vi "Morphological Segmentation.vi"() -> ()   [LabVIEW 2014]
doc: "This example demonstrates a watershed transform as part of a morphological segmentation process. First, a sample image is thesholded, and a distance transform is applied to the sample image. Next, a watershed transform is applied to the image. A threshold of the watershed image is then used to separate the particles."
uses:
  <vilib>/vision/NI_Vision_Development_Module.lvlib
panel:
  in  "Images":T1(tab)=enum."Result Image"
  out "Source Image":T2(plugin-control)
  out "Threshold Image":T2(plugin-control)
  out "Distance Image":T2(plugin-control)
  out "Watershed Image":T2(plugin-control)
  out "Result Image":T2(plugin-control)
  # "Overview: Demonstrate a segmentation using the Watershed algorithm to separate objects.\nRequirements: Vision Development Module.\nInstructions:\n1. Run the VI.\n2. Browse the different tabs to see the image after each operation."
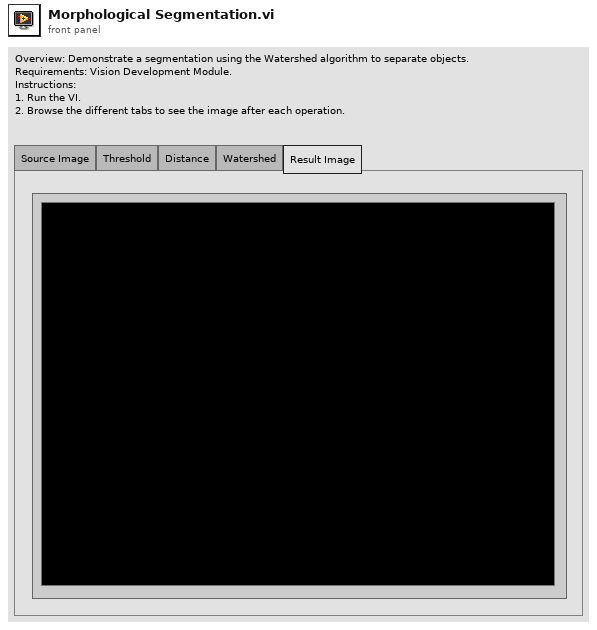
[diagram p1: front panel]
types:
  T1 = enum32{"Source Image", "Threshold", "Distance", "Watershed", "Result Image"}
  T2 = typedef "IMAQ Image.ctl" = refnum<image>
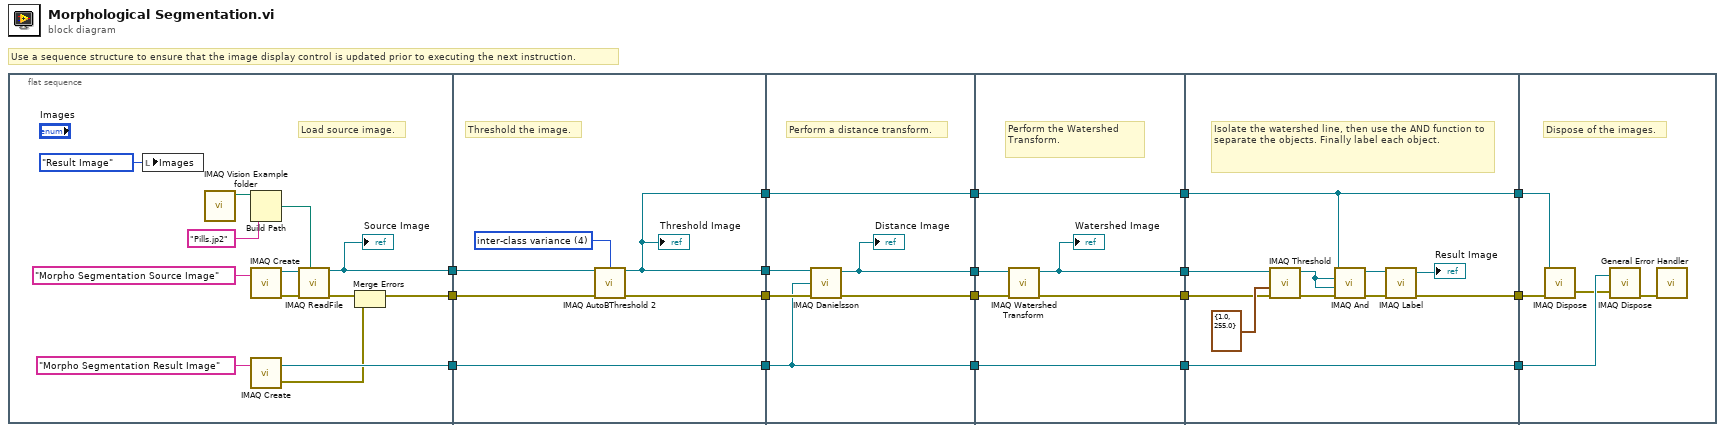
[diagram p0: block diagram]
diagram:
  # "Use a sequence structure to ensure that the image display control is updated prior to executing the next instruction."
  n1 = flat-sequence {
    tunnel: [w25] -> w18
    tunnel: [w22] -> w12
    tunnel: [w19] -> w1
    tunnel: w18 -> [w33]
    tunnel: [w35] -> w17
    tunnel: [w32] -> w16
    tunnel: [w33] -> w13
    tunnel: w12 -> [w36]
    tunnel: [w32] -> w3
    tunnel: w1 -> [w34]
    tunnel: w17 -> [w42]
    tunnel: w16 -> [w43]
    tunnel: [w41] -> w15
    tunnel: [w38] -> w14
    tunnel: w13 -> [w38]
    tunnel: [w40] -> w11
    tunnel: [w39] -> w4
    tunnel: w3 -> [w39]
    tunnel: w15 -> [w47]
    tunnel: [w45] -> w9
    tunnel: w14 -> [w49]
    tunnel: [w49] -> w8
    tunnel: w11 -> [w48]
    tunnel: [w46] -> w6
    tunnel: [w44] -> w5
    tunnel: w4 -> [w44]
    tunnel: [w54] -> w10
    tunnel: w9 -> [w58]
    tunnel: w8 -> [w56]
    tunnel: [w56] -> w7
    tunnel: w6 -> [w59]
    tunnel: w5 -> [w54]
    tunnel: [w50] -> w2
    tunnel: w10 -> [w65]
    tunnel: w7 -> [w63]
    tunnel: w2 -> [w64]
    frame #0 {
      # "Load source image."
      n2 = local write "Images"(T1."Result Image" ("Images")) -> ()
      n3 = call "IMAQ Vision Example folder.vi"() -> ("Example Image Path"=w29:path)  [unwired: 11 in]
      n4 = Build Path(base path=w29, name or relative path="Pills.jp2") -> (appended path=w24:path)
      n5 = call "IMAQ Create"("Image Name"="Morpho Segmentation Source Image") -> ("New Image"=w28:T2, "error out"=w27:errorcluster)  [unwired: 3 in, 1 out]
      n6 = call "IMAQ Create"("Image Name"="Morpho Segmentation Result Image") -> ("New Image"=w25:T2, "error out"=w20:errorcluster)  [unwired: 3 in, 1 out]
      n7 = call "IMAQ ReadFile"("File Path"=w24, "error in (no error)"=w27, "Image"=w28) -> ("error out"=w21:errorcluster, "Image Out"=w22:T2)  [unwired: 2 in, 5 out]
      "Source Image" <- w22
      n8 = Merge Errors(w21, w20) -> (w19:errorcluster)
    }
    frame #1 {
      w37 = 4 items=["clustering", "entropy", "metric", "moments", "inter-class variance"] ("Method")
      # "Threshold the image."
      n9 = call "IMAQ AutoBThreshold 2"("Image Src"=w36, "Method (clustering)"=w37, "error in (no error)"=w34) -> ("Image Dst Out"=w32:T2, "error out"=w35:errorcluster)  [unwired: 5 in, 6 out]
      "Threshold Image" <- w32
    }
    frame #2 {
      # "Perform a distance transform."
      n10 = call "IMAQ Danielsson"("error in (no error)"=w42, "Image Dst"=w38, "Image Src"=w43) -> ("error out"=w41:errorcluster, "Image Dst Out"=w40:T2)  [unwired: 1 out]
      "Distance Image" <- w40
    }
    frame #3 {
      # "Perform the Watershed Transform."
      n11 = call "IMAQ Watershed Transform"("error in (no error)"=w47, "Image Src"=w48) -> ("error out"=w45:errorcluster, "Image Dst Out"=w46:T2)  [unwired: 2 in, 6 out]
      "Watershed Image" <- w46
    }
    frame #4 {
      # "Isolate the watershed line, then use the AND function to separate the objects. Finally label each object."
      n12 = call "IMAQ Threshold"("error in (no error)"=w58, "Range"=cluster{"Lower value":sgl, "Upper value":sgl} {"Lower value"=1.0, "Upper value"=255.0}, "Image Src"=w59) -> ("error out"=w57:errorcluster, "Image Dst Out"=w55:T2)  [unwired: 3 in, 4 out]
      n13 = call "IMAQ And"("error in (no error)"=w57, "Image Src B"=w55, "Image Dst"=w55, "Image Src A"=w54) -> ("error out"=w52:errorcluster, "Image Dst Out"=w53:T2)  [unwired: 6 in]
      n14 = call "IMAQ Label"("error in (no error)"=w52, "Image Src"=w53) -> ("error out"=w50:errorcluster, "Image Dst Out"=→"Result Image":T2)  [unwired: 2 in, 1 out]
    }
    frame #5 {
      # "Dispose of the images."
      n15 = call "IMAQ Dispose"("Image"=w65, "error in (no error)"=w64) -> ("error out"=w62:errorcluster)  [unwired: 1 in, 3 out]
      n16 = call "IMAQ Dispose"("Image"=w63, "error in (no error)"=w62) -> ("error out"=w61:errorcluster)  [unwired: 1 in, 3 out]
      n17 = call <vilib>:"General Error Handler.vi"("error in (no error)"=w61) -> ()  [unwired: 10 in, 5 out]
    }
  }
